vi "tb_interleave two fft dit_host_sgl.vi"() -> ()   [LabVIEW 2011]
uses:
  <userlib>/FPGA Library/Code Development/Signal Processing/FFT Block/FFT/FFT Size.ctl
  <vilib>/Analysis/2dsp.llb/Real FFT.vi
  <vilib>/imath/engines/lvmath2/RunTimeEngine/ErrorHandling/NIMS_Finalize Error.vi
  <vilib>/imath/engines/lvmath2/RunTimeEngine/NodeEndStatement/NIMS_NodeEndStatement_Output.vi
  <instcachedir>/0/NIMS_NodeEndStatement_Output_53EC0D466D134D7ABD903AC30B43404B.lvgen/NIMS_NodeEndStatement_Output_53EC0D466D134D7ABD903AC30B43404B_000.vi
  <vilib>/imath/engines/lvmath2/RunTimeEngine/RangeToken/NIMS_Range.vi
  <instcachedir>/0/NIMS_Range_0B7635FB69F84E19AA68E7FF959DF37C.lvgen/NIMS_Range_0B7635FB69F84E19AA68E7FF959DF37C_000.vi
  <vilib>/imathl/engines/lvmath/Functions/Error Handling/Create Error.vi
  <vilib>/rvi/FXPMathLib/basic elements/FxpDiscreteDelay/XNode/nifxpmath_DiscreteDelay.xnode
  <vilib>/Analysis/NI_AALPro.lvlib
  <vilib>/Analysis/NI_AALBase.lvlib
panel:
  out "prod_fpga":cdb[](array[numeric])
  out "twiddle_labview":cdb[](array[numeric])
  out "twiddle_fpga":cdb[](array[numeric])
  out "fpga":cdb[](array[numeric])
  out "prod_labview":cdb[](array[numeric])
  out "Log Error":dbl[](graph)
  out "Error":dbl[](graph)
  out "LabVIEW FLP DIT":dbl[](graph)
  out "size(s)":i32
  out "LabVIEW FLP":dbl[](graph)
  out "FXP Coregen":dbl[](graph)
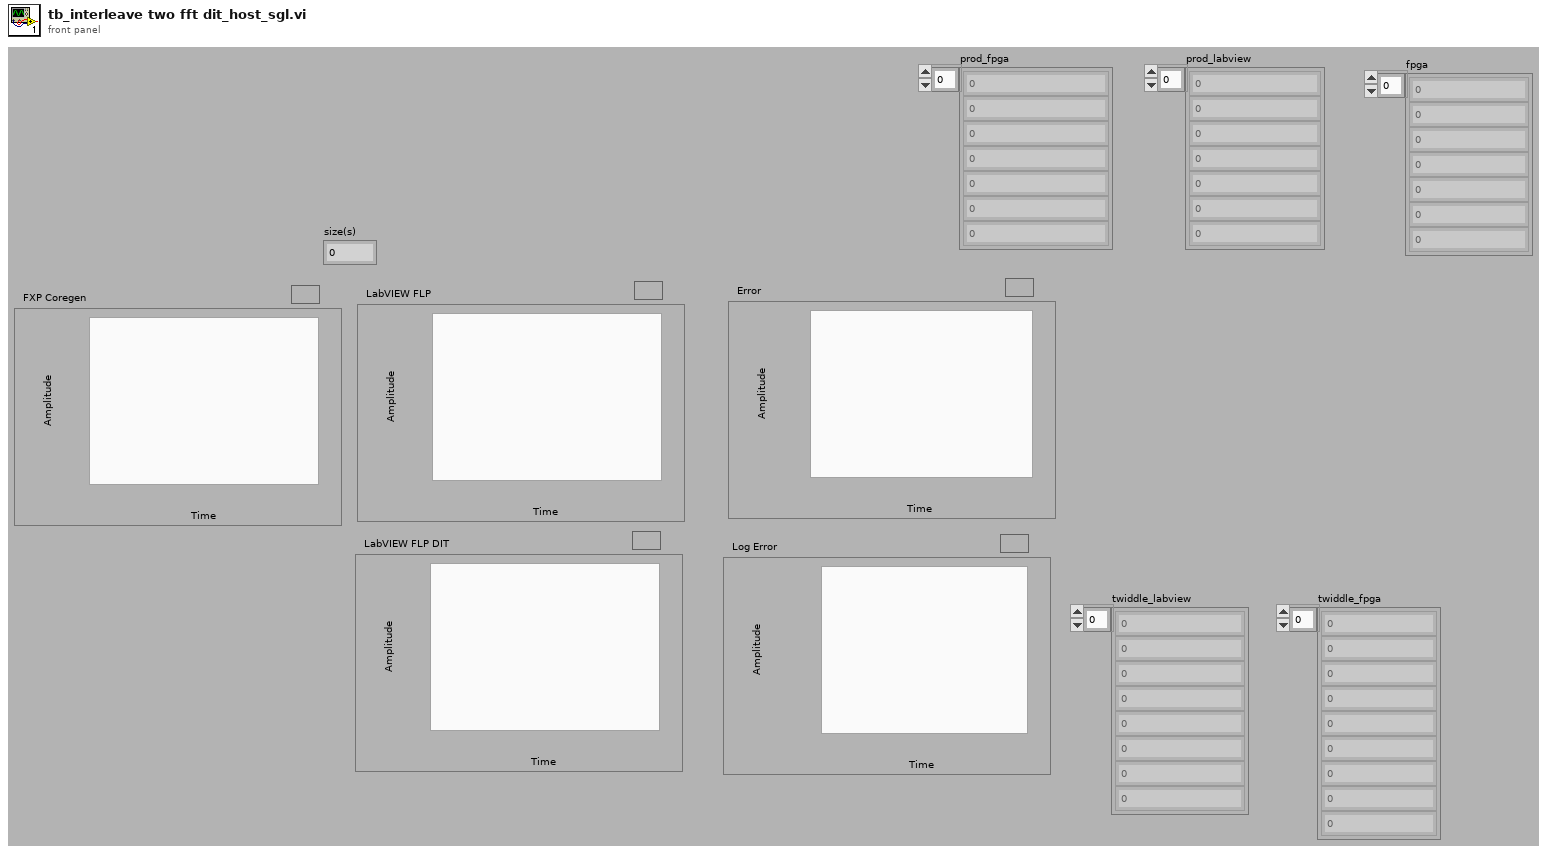
[diagram p1: front panel]
types:
  T1 = cluster{"xk_im":fxp<+,32,32>, "xk_re":fxp<+,32,32>}
  T2 = typedef "FFT Size.ctl" = enum16{"512", "1024", "2048", "4096", "8192", "16384", "32768", "65536"}
  T3 = cluster{"Yout":fxp<+,32,32>, "Xout":fxp<+,32,32>}
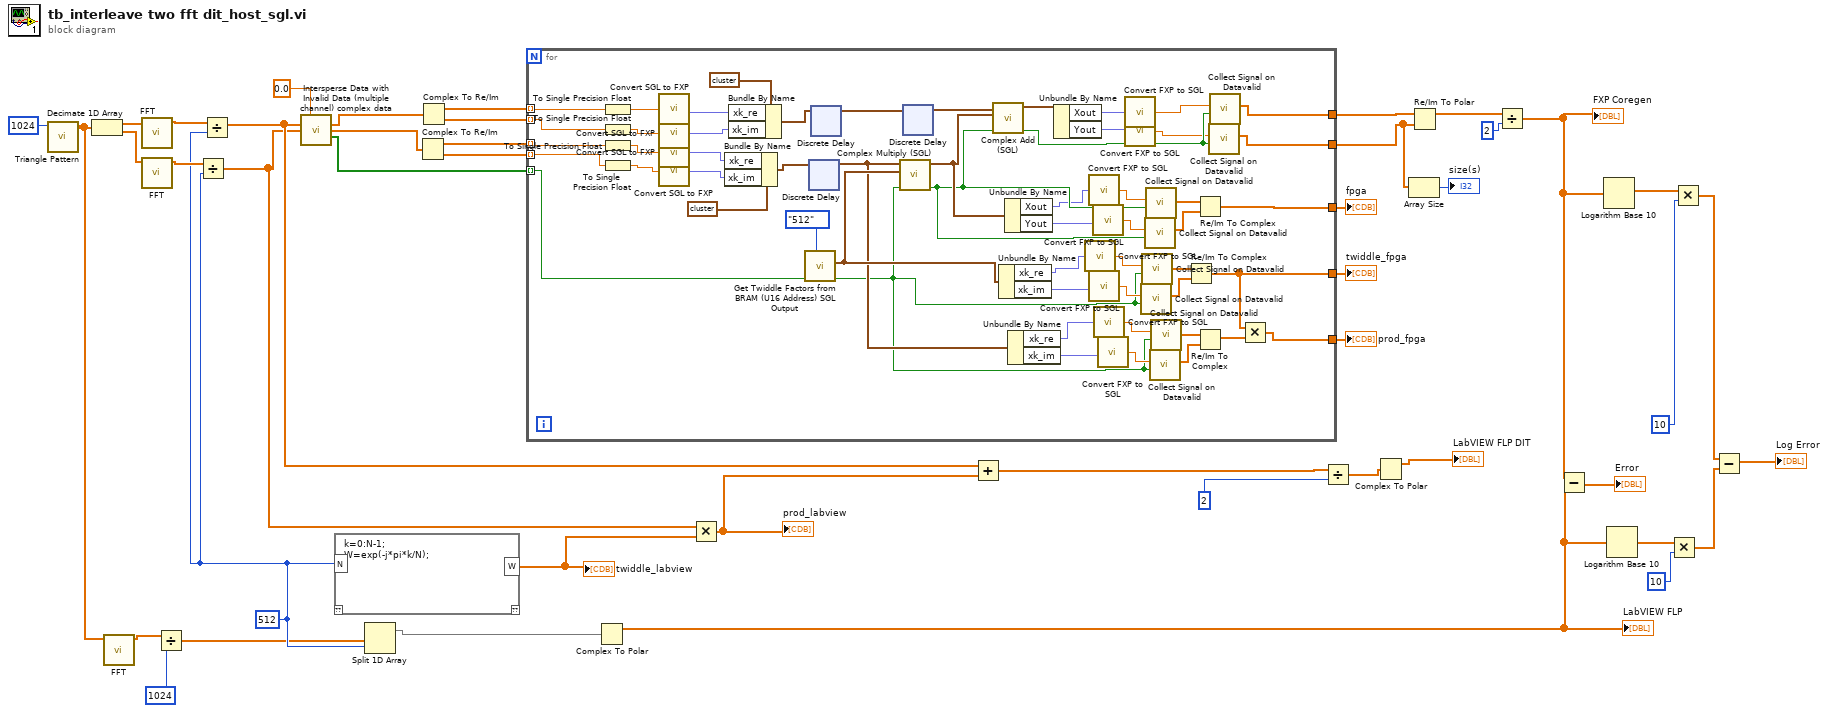
[diagram p0: block diagram]
diagram:
  w29 = 512 ("index")
  n1 = call <vilib>:"Triangle Pattern.vi"("samples"=1024) -> ("Triangle Pattern"=w38:dbl[])  [unwired: 9 in, 1 out]
  n2 = Decimate 1D Array(w38) -> (w40:dbl[], w39:dbl[])
  n3 = call-poly <vilib>:"FFT.vi"("X"=w38) -> ("FFT {X}"=w28:cdb[])  [unwired: 9 in, 1 out]
  n4 = call-poly <vilib>:"FFT.vi"("X"=w40) -> ("FFT {X}"=w31:cdb[])  [unwired: 9 in, 1 out]
  n5 = call-poly <vilib>:"FFT.vi"("X"=w39) -> ("FFT {X}"=w30:cdb[])  [unwired: 9 in, 1 out]
  n6 = Divide(x=w28, y=1024) -> (x/y=w26:cdb[])
  n7 = Divide(x=w30, y=w29) -> (x/y=w6:cdb[])
  n8 = Divide(x=w31, y=w29) -> (x/y=w19:cdb[])
  n9 = call <userlib>:"Intersperse Data with Invalid Data (multiple channel) complex data.vi"("Intersperse Ratio"=0.0, "Channel0 Input"=w19, "Channel1 Input"=w6) -> ("Channel0 Output"=w22:cdb[], "Channel1 Output"=w21:cdb[], "Data Valid"=w20:bool[])  [unwired: 10 in]
  n10 = mathscript code="k=0:N-1;\nW=exp(-j*pi*k/N);"("N"=w29) -> ("W"=w33:cdb[])  [unwired: 1 in, 1 out]
  "twiddle_labview" <- w33
  n11 = Split 1D Array(array=w26, index=w29) -> (first subarray=w36:cdb[])  [unwired: 1 out]
  n12 = Complex To Re/Im(x + iy=w21) -> (x=w42:dbl[], y=w41:dbl[])
  n13 = Complex To Re/Im(x + iy=w22) -> (x=w44:dbl[], y=w43:dbl[])
  n14 = for {
    tunnel: w44 -> [w94] mode=indexing
    tunnel: w43 -> [w91] mode=indexing
    tunnel: w42 -> [w93] mode=indexing
    tunnel: w41 -> [w92] mode=indexing
    tunnel: [w100] -> w37
    tunnel: [w99] -> w35
    tunnel: w20 -> [w95] mode=indexing
    tunnel: [w72] -> w9
    tunnel: [w51] -> w8
    tunnel: [w50] -> w7
    n15 = To Single Precision Float(number=w94) -> (single precision float=w90:sgl)
    n16 = To Single Precision Float(number=w91) -> (single precision float=w89:sgl)
    n17 = To Single Precision Float(number=w93) -> (single precision float=w88:sgl)
    n18 = To Single Precision Float(number=w92) -> (single precision float=w87:sgl)
    n19 = call <userlib>:"Convert SGL to FXP.vi"("Input"=w90) -> ("FXP Output"=w85:fxp<+,32,32>)  [unwired: 14 in]
    n20 = call <userlib>:"Convert SGL to FXP.vi"("Input"=w89) -> ("FXP Output"=w84:fxp<+,32,32>)  [unwired: 14 in]
    n21 = call <userlib>:"Convert SGL to FXP.vi"("Input"=w88) -> ("FXP Output"=w82:fxp<+,32,32>)  [unwired: 14 in]
    n22 = call <userlib>:"Convert SGL to FXP.vi"("Input"=w87) -> ("FXP Output"=w81:fxp<+,32,32>)  [unwired: 14 in]
    n23 = Bundle By Name(cluster=T1 {"xk_im"=0.0, "xk_re"=0.0} ("D"), "xk_re"=w82, "xk_im"=w81) -> (w80:T1)
    n24 = Bundle By Name(cluster=T1 {"xk_im"=0.0, "xk_re"=0.0} ("D"), "xk_re"=w85, "xk_im"=w84) -> (w79:T1)
    n25 = call <userlib>:"Get Twiddle Factors from BRAM (U16 Address) SGL Output.vi"("FFT Size"=FFT_Size."512", "Input Data Valid"=w95) -> ("Output Valid"=w53:bool, "Output"=w61:T1)  [unwired: 7 in, 1 out]
    n26 = xnode "Discrete Delay"("D"=w80) -> ("Q"=w56:T1)
    n27 = xnode "Discrete Delay"("D"=w79) -> ("Q"=w98:T1)
    n28 = call <userlib>:"Complex Multiply (SGL).vi"("Input Valid"=w53, "X2+j Y2"=w61, "X1+j Y1"=w56) -> ("Output Valid"=w75:bool, "Xout+j Yout"=w76:T3)  [unwired: 7 in]
    n29 = xnode "Discrete Delay"("D"=w98) -> ("Q"=w97:T1)
    n30 = call <userlib>:"Complex Add (SGL).vi"("Input Valid"=w75, "X2+j Y2"=w76, "X1+j Y1"=w97) -> ("Output Valid"=w77:bool, "Xout+j Yout"=w78:T3)  [unwired: 7 in]
    n31 = Unbundle By Name(w61) -> ("xk_re"=w66:fxp<+,32,32>, "xk_im"=w67:fxp<+,32,32>)
    n32 = Unbundle By Name(w76) -> ("Xout"=w69:fxp<+,32,32>, "Yout"=w68:fxp<+,32,32>)
    n33 = Unbundle By Name(w56) -> ("xk_re"=w55:fxp<+,32,32>, "xk_im"=w57:fxp<+,32,32>)
    n34 = Unbundle By Name(w78) -> ("Xout"=w49:fxp<+,32,32>, "Yout"=w48:fxp<+,32,32>)
    n35 = call <userlib>:"Convert FXP to SGL.vi"("FXP Input"=w66) -> ("Output SGL"=w65:sgl)  [unwired: 14 in]
    n36 = call <userlib>:"Convert FXP to SGL.vi"("FXP Input"=w69) -> ("Output SGL"=w70:sgl)  [unwired: 14 in]
    n37 = call <userlib>:"Convert FXP to SGL.vi"("FXP Input"=w67) -> ("Output SGL"=w64:sgl)  [unwired: 14 in]
    n38 = call <userlib>:"Convert FXP to SGL.vi"("FXP Input"=w68) -> ("Output SGL"=w71:sgl)  [unwired: 14 in]
    n39 = call <userlib>:"Convert FXP to SGL.vi"("FXP Input"=w55) -> ("Output SGL"=w54:sgl)  [unwired: 14 in]
    n40 = call <userlib>:"Convert FXP to SGL.vi"("FXP Input"=w57) -> ("Output SGL"=w58:sgl)  [unwired: 14 in]
    n41 = call <userlib>:"Convert FXP to SGL.vi"("FXP Input"=w49) -> ("Output SGL"=w46:sgl)  [unwired: 14 in]
    n42 = call <userlib>:"Convert FXP to SGL.vi"("FXP Input"=w48) -> ("Output SGL"=w47:sgl)  [unwired: 14 in]
    n43 = call <userlib>:"Collect Signal on Datavalid.vi"("Data Valid"=w53, "Input"=w64) -> ("Output"=w63:dbl[])  [unwired: 9 in]
    n44 = call <userlib>:"Collect Signal on Datavalid.vi"("Data Valid"=w53, "Input"=w65) -> ("Output"=w62:dbl[])  [unwired: 9 in]
    n45 = call <userlib>:"Collect Signal on Datavalid.vi"("Data Valid"=w75, "Input"=w71) -> ("Output"=w73:dbl[])  [unwired: 9 in]
    n46 = call <userlib>:"Collect Signal on Datavalid.vi"("Data Valid"=w75, "Input"=w70) -> ("Output"=w74:dbl[])  [unwired: 9 in]
    n47 = call <userlib>:"Collect Signal on Datavalid.vi"("Data Valid"=w53, "Input"=w58) -> ("Output"=w59:dbl[])  [unwired: 9 in]
    n48 = call <userlib>:"Collect Signal on Datavalid.vi"("Data Valid"=w53, "Input"=w54) -> ("Output"=w60:dbl[])  [unwired: 9 in]
    n49 = Re/Im To Complex(1:w63, 2:w62) -> (0:w51:cdb[])
    n50 = Re/Im To Complex(1:w73, 2:w74) -> (0:w72:cdb[])
    n51 = Re/Im To Complex(1:w59, 2:w60) -> (0:w52:cdb[])
    n52 = call <userlib>:"Collect Signal on Datavalid.vi"("Data Valid"=w77, "Input"=w47) -> ("Output"=w99:dbl[])  [unwired: 9 in]
    n53 = call <userlib>:"Collect Signal on Datavalid.vi"("Data Valid"=w77, "Input"=w46) -> ("Output"=w100:dbl[])  [unwired: 9 in]
    n54 = Multiply(x=w51, y=w52) -> (x*y=w50:cdb[])
  }
  "fpga" <- w9
  "twiddle_fpga" <- w8
  "prod_fpga" <- w7
  n55 = Complex To Polar(r * e^(i*theta)=w36) -> (r=w17:dbl[])  [unwired: 1 out]
  "LabVIEW FLP" <- w17
  n56 = Multiply(x=w6, y=w33) -> (x*y=w4:cdb[])
  "prod_labview" <- w4
  n57 = Add(x=w19, y=w4) -> (x+y=w25:cdb[])
  n58 = Divide(x=w25, y=2 ("index")) -> (x/y=w23:cdb[])
  n59 = Complex To Polar(r * e^(i*theta)=w23) -> (r=→"LabVIEW FLP DIT":dbl[])  [unwired: 1 out]
  n60 = Array Size(array=w35) -> (size(s)=→"size(s)":i32)
  n61 = Re/Im To Polar(2:w35, 3:w37) -> (1:w3:dbl[])  [unwired: 1 out]
  n62 = Divide(x=w3, y=2 ("index")) -> (x/y=w1:dbl[])
  "FXP Coregen" <- w1
  n63 = Subtract(x=w1, y=w17) -> (x-y=→"Error":dbl[])
  n64 = Logarithm Base 10(1:w1) -> (0:w16:dbl[])
  n65 = Logarithm Base 10(1:w17) -> (0:w13:dbl[])
  n66 = Multiply(x=w13, y=10) -> (x*y=w11:dbl[])
  n67 = Multiply(x=w16, y=10) -> (x*y=w12:dbl[])
  n68 = Subtract(x=w12, y=w11) -> (x-y=→"Log Error":dbl[])
